vi "WPILogOpen.vi"(8 "error in (no error)":errorcluster, 10 "loading q":refnum<queue>, 11 "File Path":path) -> (0 "error out":errorcluster, 3 "WPILog Ref":refnum<data-value>)   [LabVIEW 2020]
uses:
  Typedef/WPILibLog.ctl
  Typedef/Header.ctl
  Typedef/Entry.ctl
  Typedef/Record.ctl
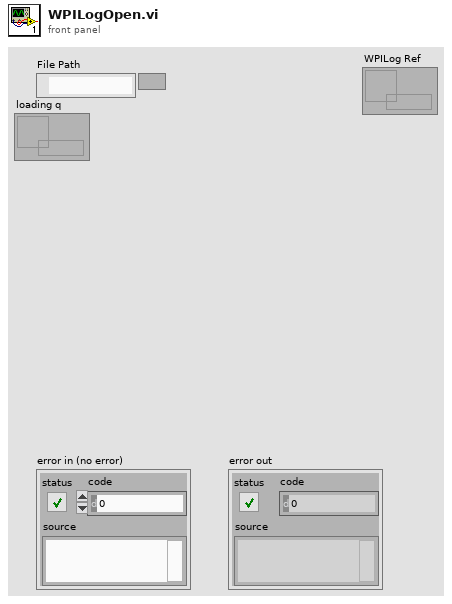
[diagram p1: front panel]
types:
  T1 = typedef "WPILibLog.ctl" = cluster{"Header":T2, "Record Start Idx":i32, "Entries":map{u32, T3}, "file ref":refnum<file>, "Finished Entries":T3[], "raw data":u8[]}
  T2 = typedef "Header.ctl" = cluster{"Header String":string, "Version":dbl, "Header Extra String Length":u32, "Header Extra String":string}
  T3 = typedef "Entry.ctl" = cluster{"ID":u32, "Records":T4[], "Finished?":bool, "Name":string, "Type":string, "Metadata":string, "RecordCnt":i32}
  T4 = typedef "Record.ctl" = cluster{"raw data":u8[], "ID":u32, "Size (bytes)":u32, "Timestamp":u64}
  T5 = enum16{"big-endian, network order", "native, host order", "little-endian"}
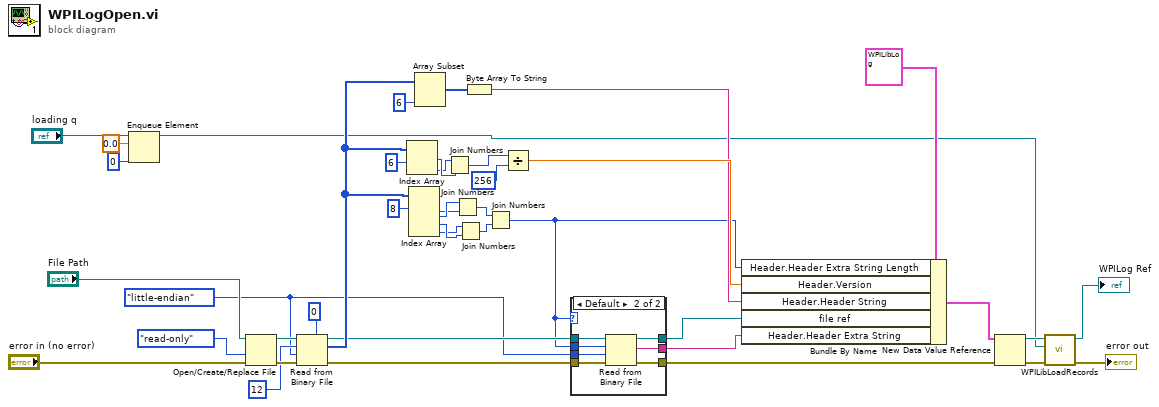
[diagram p0: block diagram]
diagram:
  w13 = T5."little-endian" ("byte order (0:big-endian, network order)")
  n1 = Enqueue Element(queue="loading q", element=0.0, timeout in ms (-1)=0) -> (queue out=w1:refnum<queue>)  [unwired: 1 in, 2 out]
  n2 = Open/Create/Replace File(file path (use dialog)="File Path", error in="error in (no error)", access (0:read/write)=enum16{"read/write", "read-only", "write-only"}."read-only") -> (refnum out=w19:refnum<file>, error out=w20:errorcluster)  [unwired: 3 in, 1 out]
  n3 = Read from Binary File(5:u8 0, 8:w20, 9:w13, 10:12 ("count (1)"), 11:w19) -> (0:w9:errorcluster, 2:w17:u8[], 3:w14:refnum<file>)  [unwired: 1 in, 1 out]
  n4 = Index Array(array=w17, index #1=6 ("index")) -> (element #1=w31:u8, element #2=w30:u8)  [unwired: 1 in]
  n5 = Index Array(array=w17, index #1=8 ("index")) -> (element #1=w33:u8, element #2=w34:u8, element #3=w36:u8, element #4=w35:u8)  [unwired: 3 in]
  n6 = Array Subset(array=w17, length=6) -> (w26:u8[])  [unwired: 1 in]
  n7 = Join Numbers(hi=w30, lo=w31) -> ((hi.lo)=w40:u16)
  n8 = Join Numbers(hi=w34, lo=w33) -> ((hi.lo)=w38:u16)
  n9 = Join Numbers(hi=w35, lo=w36) -> ((hi.lo)=w37:u16)
  n10 = Byte Array To String(unsigned byte array=w26) -> (string=w28:string)
  n11 = Join Numbers(hi=w38, lo=w37) -> ((hi.lo)=w12:u32)
  n12 = Divide(x=w40, y=u16 256 ("x")) -> (x/y=w39:dbl)
  n13 = case shown="Default" w12 {
    tunnel: [w43 w50] -> w15
    tunnel: w14 -> [w43 w49]
    tunnel: w13 -> [_ w48]
    tunnel: w12 -> [_ w47]
    tunnel: [_ w46] -> w11
    tunnel: [w42 w45] -> w10
    tunnel: w9 -> [w42 w44]
    frame ..0 {
    }
    frame Default {
      n14 = Read from Binary File(8:w44, 9:w48, 10:w47, 11:w49) -> (0:w45:errorcluster, 2:w46:string, 3:w50:refnum<file>)  [unwired: 2 in, 1 out]
    }
  }
  n15 = Bundle By Name(cluster=T1 {"Header"={"Header String"="", "Version"=0.0, "Header Extra String Length"=0, "Header Extra String"=""}, "Record Start Idx"=0, "Entries"={}, "file ref"=refnum, "Finished Entries"=[], "raw data"=[]}, "Header.Header Extra String Length"=w12, "Header.Version"=w39, "Header.Header String"=w28, "file ref"=w15, "Header.Header Extra String"=w11) -> (w24:T1)
  n16 = New Data Value Reference(data value=w24, error in=w10) -> (data value reference=w8:refnum<data-value>, error out=w7:errorcluster)
  n17 = call "WPILibLoadRecords.vi"("error in (no error)"=w7, "loading q"=w1, "Data Value Reference in"=w8) -> ("error out"=→"error out":errorcluster, "Data Value Reference out"=→"WPILog Ref":refnum<data-value>)  [unwired: 7 in]
